vi "teleop Intake subVI.vi"(9 "Buttons":bool[](array[boolean]), 10 "Axes":dbl[](array[numeric])) -> ()   [LabVIEW 2017]
uses:
  <vilib>/Rock Robotics/WPI/Solenoid/WPI_SolenoidValue.ctl
  <vilib>/Rock Robotics/WPI/Solenoid/WPI_SolenoidSetEnum.vi
  <vilib>/Rock Robotics/Network Tables/NT Read Number.vi
  <vilib>/Rock Robotics/Network Tables/NT Write Number.vi
panel:
  out "Elevation":dbl
  # "e"
  # "1. a\n2. b\n3.x \n4. y\n5. LB \n6. RB\n7. Back\n8 start\n9. LT\n10 RT"
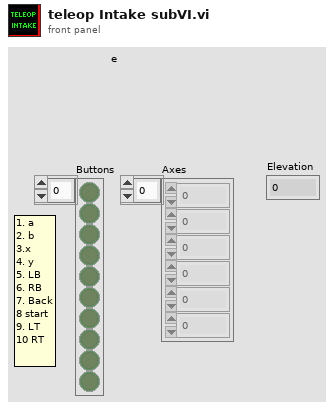
[diagram p1: front panel]
types:
  T1 = typedef "WPI_SolenoidValue.ctl" = enum16{"Off", "On", "Forward", "Reverse"}
  T2 = typedef "WPI_SolenoidDevRef.ctl" = cluster{"DevStatus":errorcluster, "Pneumatics Control Module":u8, "Forward Solenoid Channel":T3, "Reverse Solenoid Channel":T3}
  T3 = typedef "WPI_SolenoidChannel.ctl" = enum8{"Solenoid 0", "Solenoid 1", "Solenoid 2", "Solenoid 3", "Solenoid 4", "Solenoid 5", "Solenoid 6", "Solenoid 7", "Invalid"}
  T4 = typedef "WPI_MotorControlDeviceRef.ctl" = cluster{"DeviceStatus":errorcluster, "Type":T5, "PWM":cluster{"PWM Channel":T6, "DeadBand":T7}, "CAN":cluster{"Device Number":u8, "SetOutput VI Ref":variant, "GetOutput VI Ref":variant, "Enable VI Ref":variant, "Disable VI Ref":variant, "Data":variant}, "Invert":bool, "DIO PWM":cluster{"PWM \"Enable\" Channel":T6, "DIOChannel":T8, "PWM Rate":dbl}}
  T5 = typedef "WPI_MotorControlType.ctl" = enum16{"PWM", "CAN", "DIO PWM"}
  T6 = typedef "FPGA_DIOPWMChannel.ctl" = enum8{"PWM 0", "PWM 1", "PWM 2", "PWM 3", "PWM 4", "PWM 5", "PWM 6", "PWM 7", "PWM 8", "PWM 9", "PWM MXP 0", "PWM MXP 1", "PWM MXP 2", "PWM MXP 3", "PWM MXP 4", "PWM MXP 5", "PWM MXP 6", "PWM MXP 7", "PWM MXP 8", "PWM MXP 9", "Invalid"}
  T7 = typedef "WPI_PWMDeadband.ctl" = cluster{"Name":string, "maxPositivePwm":i32, "minPositivePwm":i32, "centerPwm":i32, "maxNegativePwm":i32, "minNegativePwm":i32, "angularRange":u16}
  T8 = typedef "FPGA_DIOChannel.ctl" = enum8{"DIO 0", "DIO 1", "DIO 2", "DIO 3", "DIO 4", "DIO 5", "DIO 6", "DIO 7", "DIO 8", "DIO 9", "DIO MXP 0", "DIO MXP 1", "DIO MXP 2", "DIO MXP 3", "DIO MXP 4", "DIO MXP 5", "DIO MXP 6", "DIO MXP 7", "DIO MXP 8", "DIO MXP 9", "DIO MXP 10", "DIO MXP 11", "DIO MXP 12", "DIO MXP 13", "DIO MXP 14", "DIO MXP 15", "SPI Port CS1", "SPI Port CS2", "SPI Port CS3", "SPI Port MISO", "SPI Port MOSI", "Invalid"}
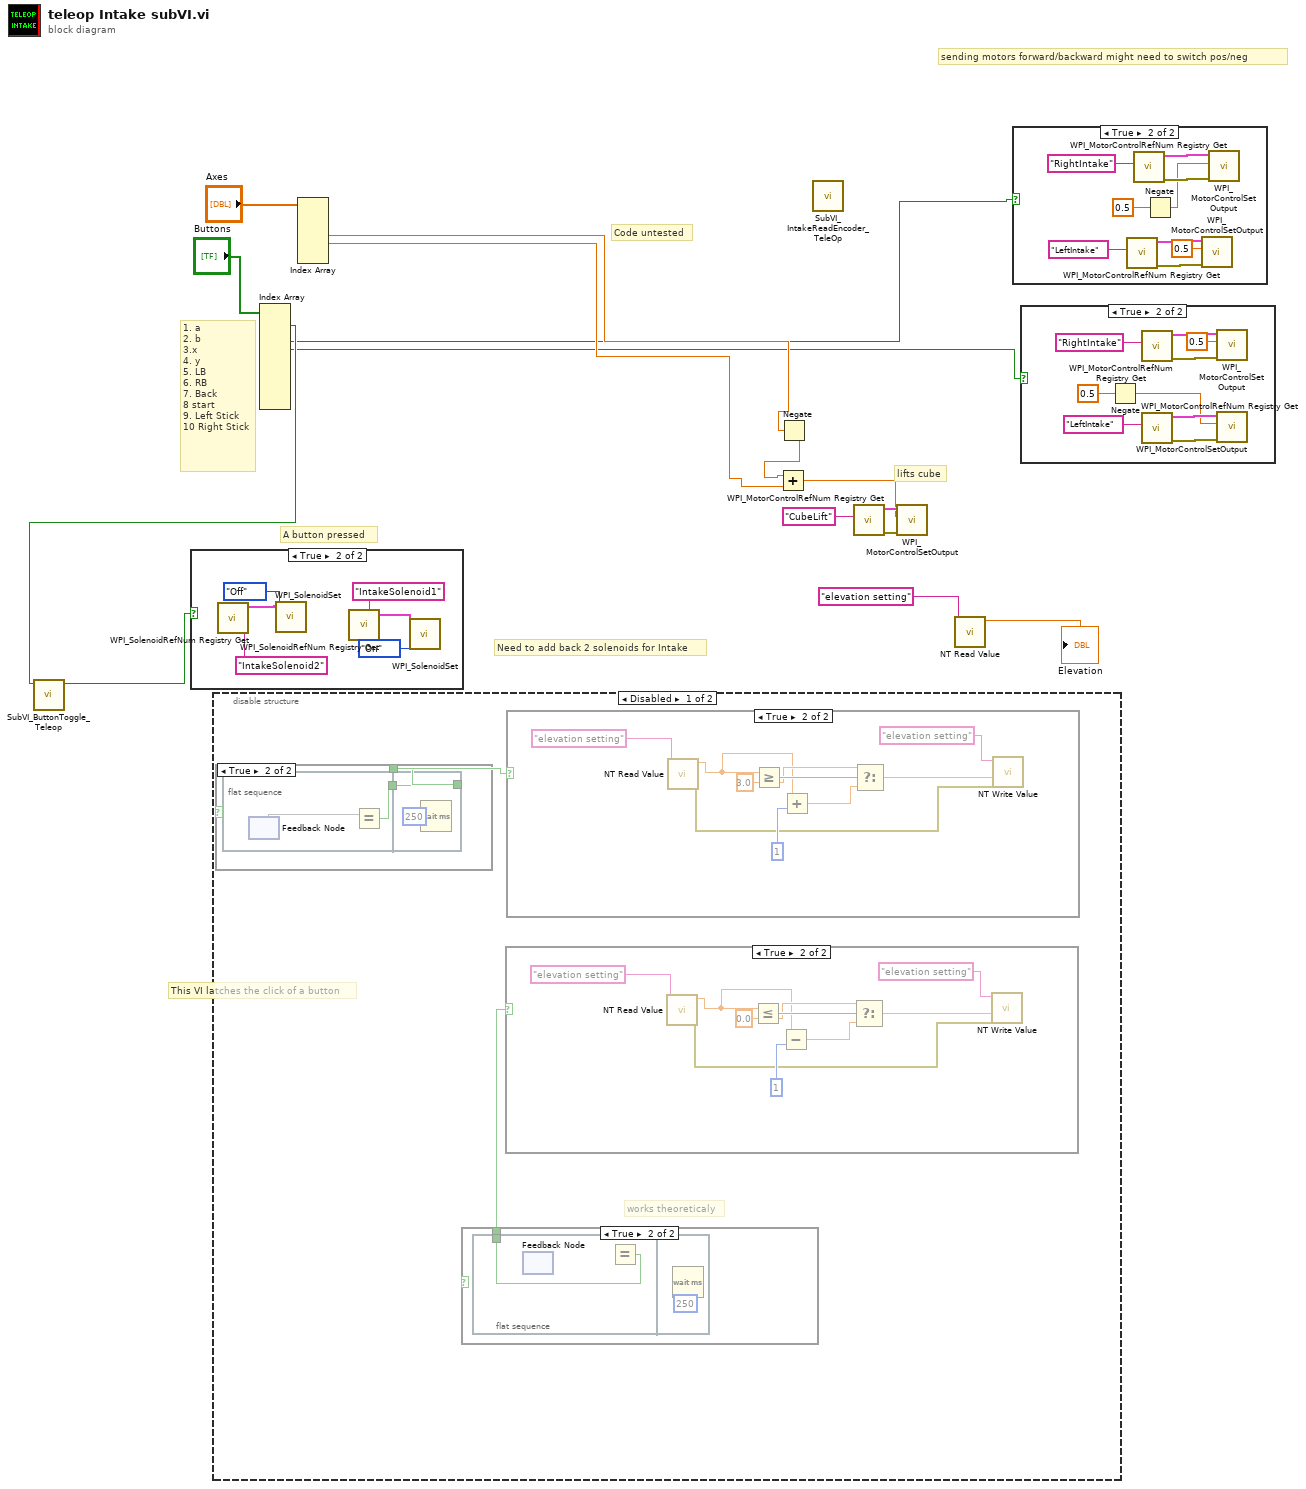
[diagram p0: block diagram]
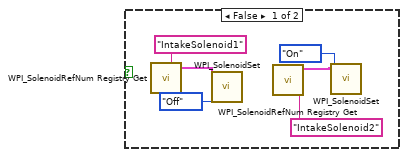
[diagram p4: hidden frame]
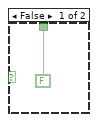
[diagram p5: hidden frame]
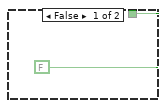
[diagram p8: hidden frame]
diagram:
  # "This VI latches the click of a button"
  # "A button pressed"
  # "lifts cube"
  # "sending motors forward/backward might need to switch pos/neg"
  # "Need to add back 2 solenoids for Intake"
  # "Code untested"
  # "1. a\n2. b\n3.x \n4. y\n5. LB \n6. RB\n7. Back\n8 start\n9. Left Stick\n10 Right Stick"
  n1 = disable-structure shown="Disabled" {
    frame Disabled {
      # "works theoreticaly"
      n2 = case shown="True" {
        selector: _ -> [_ _]
        tunnel: [FALSE w42] -> w16
        frame False {
        }
        frame True {
          n3 = flat-sequence {
            tunnel: [w43] -> w41
            tunnel: [w46] -> w42
            tunnel: w41 -> [w46]
            frame #0 {
              n4 = feedback #1() -> (w44)  [unwired: 1 in]
              n5 = feedback-in #1() -> ()  [unwired: 1 out]
              n6 = Equal?(y=w44) -> (x = y?=w43:bool)  [unwired: 1 in]
            }
            frame #1 {
              n7 = Wait (ms)(milliseconds to wait=u32 250) -> ()  [unwired: 1 out]
            }
          }
        }
      }
      n8 = case shown="True" {
        selector: _ -> [_ _]
        tunnel: [FALSE w19] -> w17
        frame False {
        }
        frame True {
          n9 = flat-sequence {
            tunnel: [w20] -> w19
            frame #0 {
              n10 = feedback #2() -> ()  [unwired: 2 in]
              n11 = feedback-in #2() -> ()  [unwired: 1 out]
              n12 = Equal?() -> (x = y?=w20:bool)  [unwired: 2 in]
            }
            frame #1 {
              n13 = Wait (ms)(milliseconds to wait=u32 250 ("millisecond timer value")) -> ()  [unwired: 1 out]
            }
          }
        }
      }
      n14 = case shown="True" w17 {
        frame False {
        }
        frame True {
          w28 = 0.0 ("y")
          n15 = call-poly <vilib>:"NT Read Value.vi"("Name"="elevation setting") -> ("error out"=w23:errorcluster, "Numeric"=w26:dbl)  [unwired: 9 in]
          n16 = Less Or Equal?(x=w26, y=w28) -> (x <= y?=w29:bool)
          n17 = Subtract(x=w26, y=1) -> (x-y=w27:dbl)
          n18 = Select(t=w28, s=w29, f=w27) -> (s? t:f=w22:dbl)
          n19 = call-poly <vilib>:"NT Write Value.vi"("error in"=w23, "Numeric"=w22, "Name"="elevation setting") -> ()  [unwired: 8 in, 1 out]
        }
      }
      n20 = case shown="True" w16 {
        frame False {
        }
        frame True {
          w37 = 3.0 ("y")
          n21 = call-poly <vilib>:"NT Read Value.vi"("Name"="elevation setting") -> ("error out"=w31:errorcluster, "Numeric"=w35:dbl)  [unwired: 9 in]
          n22 = Greater Or Equal?(x=w35, y=w37) -> (x >= y?=w38:bool)
          n23 = Add(x=w35, y=1) -> (x+y=w36:dbl)
          n24 = Select(t=w37, s=w38, f=w36) -> (s? t:f=w32:dbl)
          n25 = call-poly <vilib>:"NT Write Value.vi"("error in"=w31, "Numeric"=w32, "Name"="elevation setting") -> ()  [unwired: 8 in, 1 out]
        }
      }
    }
    frame Enabled {
    }
  }
  n26 = Index Array(array="Buttons") -> (element #1=w8:bool, element #3=w2:bool, element #4=w1:bool)  [unwired: 11 in, 8 out]
  n27 = call "SubVI_ButtonToggle_Teleop.vi"("Boolean in"=w8) -> ("Boolean out"=w7:bool)  [unwired: 10 in]
  n28 = case shown="True" w7 {
    frame False {
      n29 = call <vilib>:"WPI_SolenoidRefNum Registry Get.vi"("refnum name"="IntakeSolenoid1") -> ("SolenoidDevRef"=w52:T2)  [unwired: 9 in, 1 out]
      n30 = call-poly <vilib>:"WPI_SolenoidSet.vi"("Value"=WPI_SolenoidValue."Off", "SolenoidDevRef"=w52) -> ()  [unwired: 8 in, 2 out]
      n31 = call <vilib>:"WPI_SolenoidRefNum Registry Get.vi"("refnum name"="IntakeSolenoid2") -> ("SolenoidDevRef"=w49:T2)  [unwired: 9 in, 1 out]
      n32 = call-poly <vilib>:"WPI_SolenoidSet.vi"("Value"=WPI_SolenoidValue."On", "SolenoidDevRef"=w49) -> ()  [unwired: 8 in, 2 out]
    }
    frame True {
      n33 = call <vilib>:"WPI_SolenoidRefNum Registry Get.vi"("refnum name"="IntakeSolenoid2") -> ("SolenoidDevRef"=w58:T2)  [unwired: 9 in, 1 out]
      n34 = call-poly <vilib>:"WPI_SolenoidSet.vi"("Value"=WPI_SolenoidValue."Off", "SolenoidDevRef"=w58) -> ()  [unwired: 8 in, 2 out]
      n35 = call <vilib>:"WPI_SolenoidRefNum Registry Get.vi"("refnum name"="IntakeSolenoid1") -> ("SolenoidDevRef"=w55:T2)  [unwired: 9 in, 1 out]
      n36 = call-poly <vilib>:"WPI_SolenoidSet.vi"("Value"=WPI_SolenoidValue."On", "SolenoidDevRef"=w55) -> ()  [unwired: 8 in, 2 out]
    }
  }
  n37 = Index Array(array="Axes") -> (element #3=w5:dbl, element #4=w3:dbl)  [unwired: 6 in, 4 out]
  n38 = Negate(x=w5) -> (-x=w4:dbl)
  n39 = Add(x=w4, y=w3) -> (x+y=w6:dbl)
  n40 = call "SubVI_IntakeReadEncoder_TeleOp.vi"() -> ()  [unwired: 12 in]
  n41 = call <vilib>:"WPI_MotorControlRefNum Registry Get.vi"("refnum name"="CubeLift") -> ("error out"=w14:errorcluster, "MotorControlDevRef"=w13:T4)  [unwired: 9 in]
  n42 = call <vilib>:"WPI_MotorControlSetOutput.vi"("error in (no error)"=w14, "Output"=w6, "MotorControlDevRef"=w13) -> ()  [unwired: 6 in, 3 out]
  n43 = call-poly <vilib>:"NT Read Value.vi"("Name"="elevation setting") -> ("Numeric"=→"Elevation":dbl)  [unwired: 9 in, 1 out]
  n44 = case shown="True" w2 {
    frame False {
    }
    frame True {
      n45 = call <vilib>:"WPI_MotorControlRefNum Registry Get.vi"("refnum name"="LeftIntake") -> ("error out"=w67:errorcluster, "MotorControlDevRef"=w65:T4)  [unwired: 9 in]
      n46 = call <vilib>:"WPI_MotorControlRefNum Registry Get.vi"("refnum name"="RightIntake") -> ("error out"=w66:errorcluster, "MotorControlDevRef"=w64:T4)  [unwired: 9 in]
      n47 = Negate(x=0.5) -> (-x=w60:dbl)
      n48 = call <vilib>:"WPI_MotorControlSetOutput.vi"("error in (no error)"=w67, "Output"=0.5, "MotorControlDevRef"=w65) -> ()  [unwired: 6 in, 3 out]
      n49 = call <vilib>:"WPI_MotorControlSetOutput.vi"("error in (no error)"=w66, "Output"=w60, "MotorControlDevRef"=w64) -> ()  [unwired: 6 in, 3 out]
    }
  }
  n50 = case shown="True" w1 {
    frame False {
    }
    frame True {
      n51 = Negate(x=0.5) -> (-x=w69:dbl)
      n52 = call <vilib>:"WPI_MotorControlRefNum Registry Get.vi"("refnum name"="RightIntake") -> ("error out"=w75:errorcluster, "MotorControlDevRef"=w73:T4)  [unwired: 9 in]
      n53 = call <vilib>:"WPI_MotorControlRefNum Registry Get.vi"("refnum name"="LeftIntake") -> ("error out"=w76:errorcluster, "MotorControlDevRef"=w74:T4)  [unwired: 9 in]
      n54 = call <vilib>:"WPI_MotorControlSetOutput.vi"("error in (no error)"=w75, "Output"=0.5, "MotorControlDevRef"=w73) -> ()  [unwired: 6 in, 3 out]
      n55 = call <vilib>:"WPI_MotorControlSetOutput.vi"("error in (no error)"=w76, "Output"=w69, "MotorControlDevRef"=w74) -> ()  [unwired: 6 in, 3 out]
    }
  }
